vi "RFSG Frequency Sweep Test Signal.vi"(8 "error in (no error)":errorcluster, 9 "End Frequency (Hz)":dbl=5000000000.0 format="%#.3p", 10 "Start Frequency (Hz)":dbl=990000000.0 format="%#.3p", 11 "Resource Name":refnum<k15>="RFSG") -> (0 "error out":errorcluster)   [LabVIEW 2017]
doc: "Demonstrates how to generate a frequency sweep at a specified power level."
uses:
  <vilib>/Utility/error.llb/DialogType.ctl
  <vilib>/Analysis/1siggen.llb/Ramp Pattern by Delta.vi
  Instance           4 28Saved   RFSG Frequency Sweep .vi
  <vilib>/Analysis/NI_AALBase.lvlib
panel:
  out "samples":i32
  in  "Dwell in Each Step (s)":dbl=0.001 format="%#.6p"
  in  "Spacing (Hz)":dbl=100000000.0 format="%#_6p"
  in  "Power Level (dBm)":dbl=-10.0 format="%.2f"
  in  "Stop":bool
  out "Current Frequency (Hz)":dbl format="%#_7p"
  # "Overview: Demonstrates how to generate a frequency sweep at a specified power level.\nRequirements: NI-RFSG\nInstructions:\n1. Change the Resource Name to your device.\n2. Run the VI.\n3. Click Stop to stop the VI."
  # "Frequency Sweep Parameters"
  # "In order to configure new settings you must stop the VI using \nthe Stop button and then run the example with the new settings."
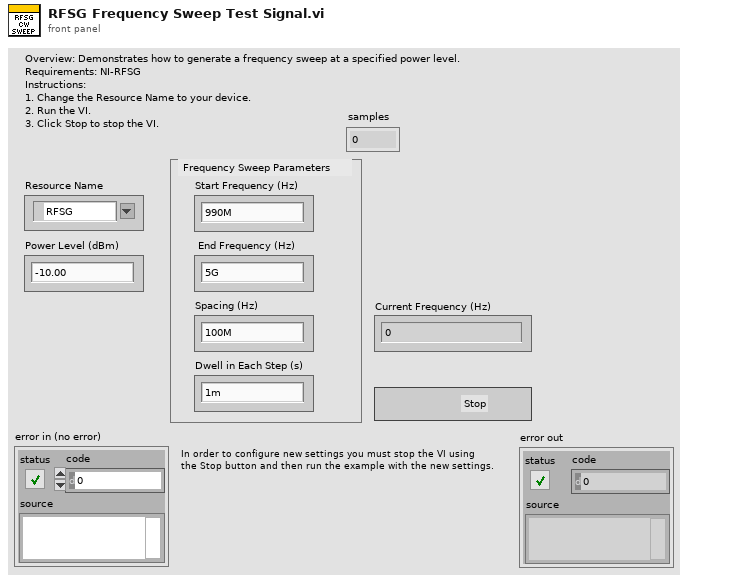
[diagram p1: front panel]
types:
  T1 = typedef "DialogType.ctl" = u16
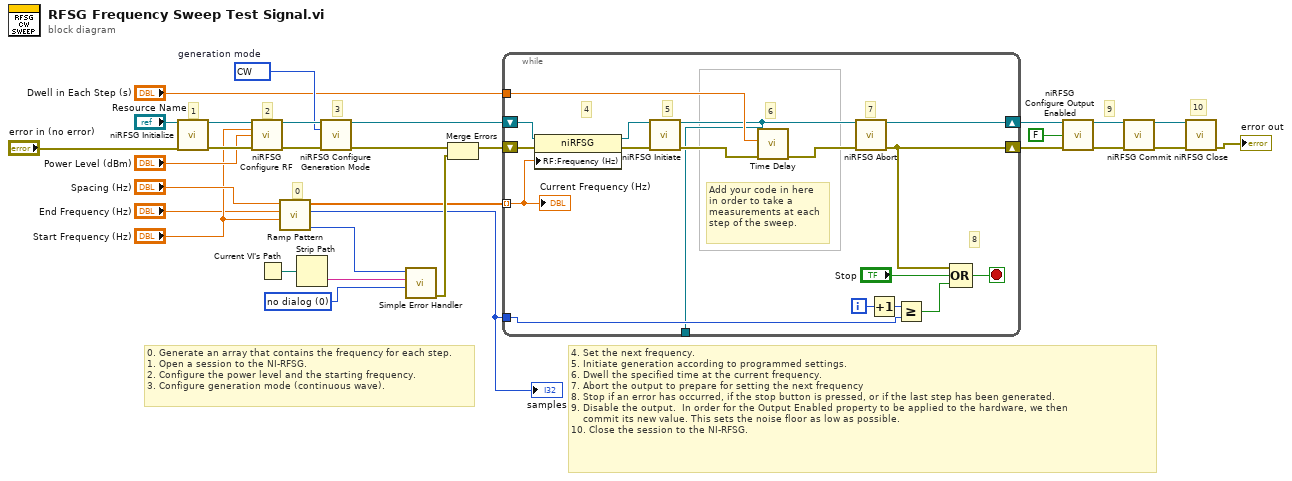
[diagram p0: block diagram]
diagram:
  w10 = 1000 items=["CW"=1000, "Arb Waveform"=1001, "Script"=1002]  # generation mode
  w27 = T1 0 items=["no dialog", "OK message", "continue or stop message", "OK message + warnings", "continue/stop + warnings"] ("type of dialog (OK msg:1)")
  # "9"
  # "3"
  # "0"
  # "4. Set the next frequency.\n5. Initiate generation according to programmed settings. \n6. Dwell the specified time at the current frequency.\n7. Abort the output to prepare for setting the next frequency \n8. Stop if an error has occurred, if the stop button is pressed, or if the last step has been generated.\n9. Disable the output.  In order for the Output Enabled property to be applied to the hardware, we then\n    commit its new value. This sets the noise floor as low as possible.  \n10. Close the session to the NI-RFSG."
  # "10"
  # "2"
  # "1"
  # "0. Generate an array that contains the frequency for each step.\n1. Open a session to the NI-RFSG.\n2. Configure the power level and the starting frequency.\n3. Configure generation mode (continuous wave)."
  n1 = call <instrlib>:"niRFSG Initialize.vi"("resource name"="Resource Name", "error in"="error in (no error)") -> ("instrument handle"=w25:refnum<k15>, "error out"=w26:errorcluster)  [unwired: 12 in]
  n2 = call <instrlib>:"niRFSG Configure RF.vi"("instrument handle"=w25, "frequency (Hz)"="Start Frequency (Hz)", "power level (dBm)"="Power Level (dBm)", "error in"=w26) -> ("instrument handle out"=w13:refnum<k15>, "error out"=w12:errorcluster)  [unwired: 10 in]
  n3 = Current VI's Path() -> (path=w30:path)
  n4 = call-poly <vilib>:"Ramp Pattern.vi"("start"="Start Frequency (Hz)", "end"="End Frequency (Hz)", "delta"="Spacing (Hz)") -> ("error"=w28:i32, "samples"=w2:i32, "Ramp Pattern"=w23:dbl[])  [unwired: 6 in]
  "samples" <- w2
  n5 = Strip Path(path=w30) -> (name=w29:string)  [unwired: 1 out]
  n6 = call <instrlib>:"niRFSG Configure Generation Mode.vi"("instrument handle"=w13, "generation mode"=w10, "error in"=w12) -> ("instrument handle out"=w1:refnum<k15>, "error out"=w11:errorcluster)  [unwired: 11 in]
  n7 = call <vilib>:"Simple Error Handler.vi"("error code (no error:0)"=w28, "error source (\" \")"=w29, "type of dialog (OK msg:1)"=w27) -> ("error out"=w24:errorcluster)  [unwired: 2 in, 4 out]
  n8 = Merge Errors(w11, w24) -> (w22:errorcluster)
  n9 = while {
    shift-right: [w33] -> w19
    shift-left: w22 -> [w45]
    tunnel: "Dwell in Each Step (s)" -> [w42]
    shift-right: [w35] -> w20
    shift-left: w1 -> [w43]
    tunnel: w23 -> [w41] mode=indexing
    tunnel: w2 -> [w32]
    tunnel: [w31] -> _
    i -> [w40]
    stop <- w47 stop-if-true
    # "7"
    # "4"
    # "Add your code in here\nin order to take a\nmeasurements at each\nstep of the sweep."
    # "8"
    # "6"
    # "5"
    n10 = property class="niRFSG"(reference=w43, error in=w45, "RF:Frequency (Hz)"=w41) -> (reference out=w36:refnum<k15>, error out=w38:errorcluster)
    n11 = call <instrlib>:"niRFSG Initiate.vi"("instrument handle"=w36, "error in"=w38) -> ("instrument handle out"=w31:refnum<k15>, "error out"=w37:errorcluster)  [unwired: 12 in]
    n12 = call "Time Delay"("error in (no error)"=w37, "Delay Time (s)"=w42) -> ("error out"=w34:errorcluster)  [unwired: 9 in]
    n13 = call <instrlib>:"niRFSG Abort.vi"("instrument handle"=w31, "error in"=w34) -> ("instrument handle out"=w35:refnum<k15>, "error out"=w33:errorcluster)  [unwired: 12 in]
    n14 = Increment(x=w40) -> (x+1=w39:i32)
    n15 = Greater Or Equal?(x=w39, y=w32) -> (x >= y?=w46:bool)
    n16 = Compound Arithmetic op=OR(w33, "Stop", w46) -> (w47:bool)
    "Current Frequency (Hz)" <- w41
  }
  n17 = call <instrlib>:"niRFSG Configure Output Enabled.vi"("instrument handle"=w20, "output enabled"=FALSE ("output enable"), "error in"=w19) -> ("instrument handle out"=w18:refnum<k15>, "error out"=w17:errorcluster)  [unwired: 11 in]
  n18 = call <instrlib>:"niRFSG Commit.vi"("instrument handle"=w18, "error in"=w17) -> ("instrument handle out"=w16:refnum<k15>, "error out"=w15:errorcluster)  [unwired: 12 in]
  n19 = call <instrlib>:"niRFSG Close.vi"("instrument handle"=w16, "error in"=w15) -> ("error out"=→"error out":errorcluster)  [unwired: 13 in]
